vi "ds get docked module id.vi"(10 "dest":u32, 11 "device_handle":u32) -> (1 "function return":i32, 2 "dest out":u32, 3 "device_handle out":u32)   [LabVIEW 2019, in "apdm.lvlib"]
doc: "APDM_EXPORT int apdm_ds_get_docked_module_id(apdm_device_handle_t device_handle, uint32_t *dest);"
uses:
  apdm.lvlib
  Lee Lab/CP FES Walking 2018/Code/Working/LabVIEW/apdm.dll
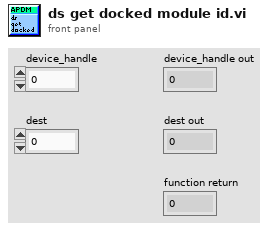
[diagram p1: front panel]
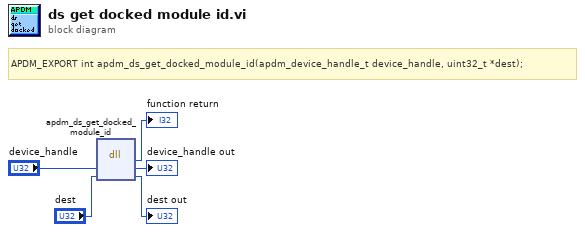
[diagram p0: block diagram]
diagram:
  # "APDM_EXPORT int apdm_ds_get_docked_module_id(apdm_device_handle_t device_handle, uint32_t *dest);"
  n1 = dll-call lib="C:/Users/jfalesi/Dropbox/Lee Lab/CP FES Walking 2018/Code/Working/LabVIEW/apdm.*" fn="apdm_ds_get_docked_module_id"("device_handle"="device_handle", "dest"="dest") -> (→"function return":i32, "device_handle"=→"device_handle out":u32, "dest"=→"dest out":u32)  [unwired: 3 in, 2 out]
